vi "Panel temperatury.vi"() -> ()   [LabVIEW 2022 SP3]
panel:
  out "String":string
  out "Meter":dbl(knob) scale=30.0..130.0
  in  "Boolean":bool
  in  "stop":bool
  out "Numer iteracji":i32
  out "Low":bool
  out "High":bool
  out "Thermometer":dbl(slide) scale=35.0..44.0
  in  "Knob 2":dbl(knob) scale=35.0..44.0
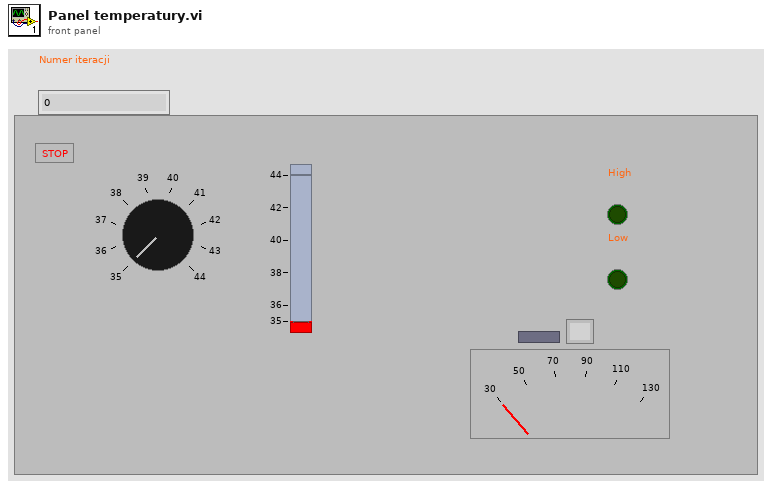
[diagram p1: front panel]
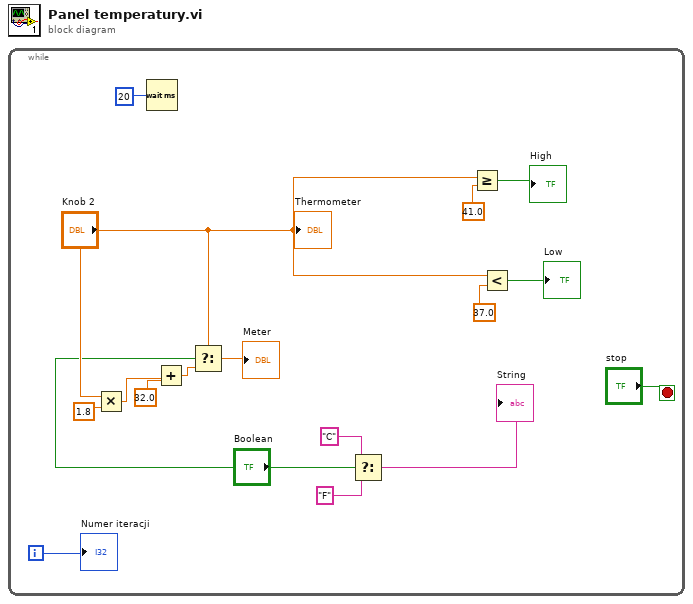
[diagram p0: block diagram]
diagram:
  n1 = while {
    i -> [w13]
    stop <- "stop" stop-if-true
    n2 = Multiply(x="Knob 2", y=1.8) -> (x*y=w6:dbl)
    n3 = Wait (ms)(milliseconds to wait=u32 20 ("millisecond timer value")) -> ()  [unwired: 1 out]
    n4 = Add(x=w6, y=32.0) -> (x+y=w5:dbl)
    n5 = Select(t="Knob 2", s="Boolean", f=w5) -> (s? t:f=→"Meter":dbl)
    n6 = Select(t="C", s="Boolean", f="F") -> (s? t:f=→"String":string)
    n7 = Greater Or Equal?(x="Knob 2", y=41.0 ("Numeric")) -> (x >= y?=→"High":bool)
    n8 = Less?(x="Knob 2", y=37.0) -> (x < y?=→"Low":bool)
    "Thermometer" <- "Knob 2"
    "Numer iteracji" <- w13
  }
